vi "struck to array.vi"(10 "Task Info":T1={"Accele Task"=[], "Simulate"=FALSE, "采样率"={"AISampleRate"=10123, "CouplingType"=10000, "Butter"=1000}, "Trig"={"PreTrigCNT"=0, "TriggerMode"=enum."中间触发", "TriggerSource"=enum."软件触发", "ATRTriggerChannel"=enum."通道0", "TriggerDir"=enum."下降沿触发", "TrigLevelVolt"=0.0, "bAvailableTrig"=FALSE}, "clock"={"EN"=FALSE, "clocksource"=enum."内部时钟", "outclocksource"=enum."Trig0"}, "delay(S)"=0.0} {"采样率"."CouplingType" items=["直流耦合", "交流耦合"]}) -> (2 "array":i32[](array[numeric]))   [LabVIEW 2009]
uses:
  Ctrls/Task Info.ctl
  Ctrls/Acceleration Channel Config_Ctrls-某型振动实验台测试系统.ctl
  Ctrls/Sample Information.ctl
  Ctrls/Trig.ctl
  Ctrls/clock.ctl
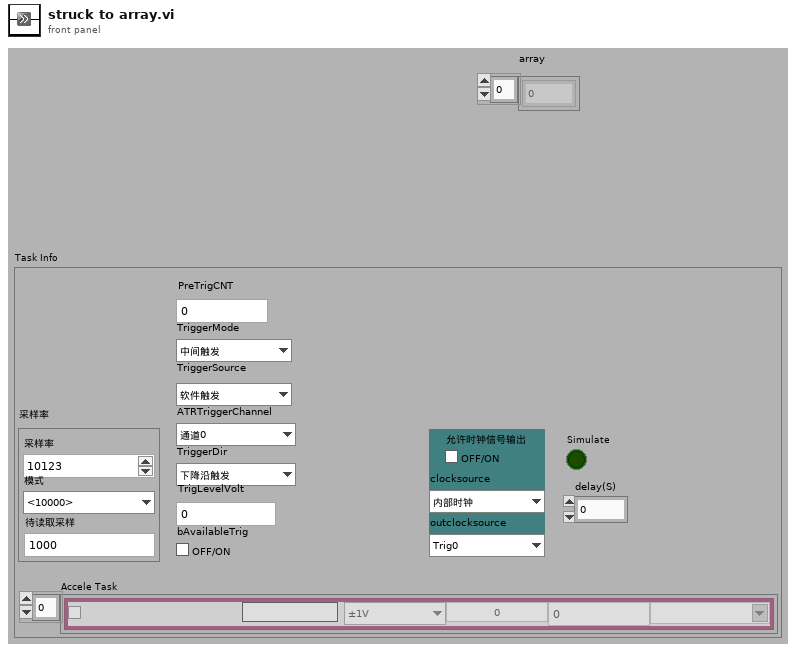
[diagram p1: front panel]
types:
  T1 = typedef "Task Info.ctl" = cluster{"Accele Task":T2[], "Simulate":bool, "采样率":T3, "Trig":T4, "clock":T5, "delay(S)":dbl}
  T2 = typedef "Acceleration Channel Config_Ctrls-某型振动实验台测试系统.ctl" = cluster{"Enable":bool, "Name":string, "range":enum16{"±1V", "±5V"}, "SensValue":dbl, "PhysicalName":string, "off":dbl, "Sensunits":string}
  T3 = typedef "Sample Information.ctl" = cluster{"AISampleRate":i32, "CouplingType":i32, "Butter":i32}
  T4 = typedef "Trig.ctl" = cluster{"PreTrigCNT":i32, "TriggerMode":enum16{"中间触发", "后触发", "预触发", "硬件延时触发"}, "TriggerSource":enum16{"软件触发", "DTR信号源", "ATR信号源", "Triger信号触发"}, "ATRTriggerChannel":enum16{"通道0", "通道1", "通道2", "通道3"}, "TriggerDir":enum16{"下降沿触发", "上升沿触发", "上下边没均触发"}, "TrigLevelVolt":sgl, "bAvailableTrig":bool}
  T5 = typedef "clock.ctl" = cluster{"EN":bool, "clocksource":enum16{"内部时钟", "外部时钟"}, "outclocksource":enum16{"Trig0", "Trig1", "Trig2", "Trig3", "Trig4", "Trig5", "Trig6", "Trig7", "PXI_STAR"}}
  T6 = enum16{"Trig0", "Trig1", "Trig2", "Trig3", "Trig4", "Trig5", "Trig6", "Trig7", "PXI_STAR"}
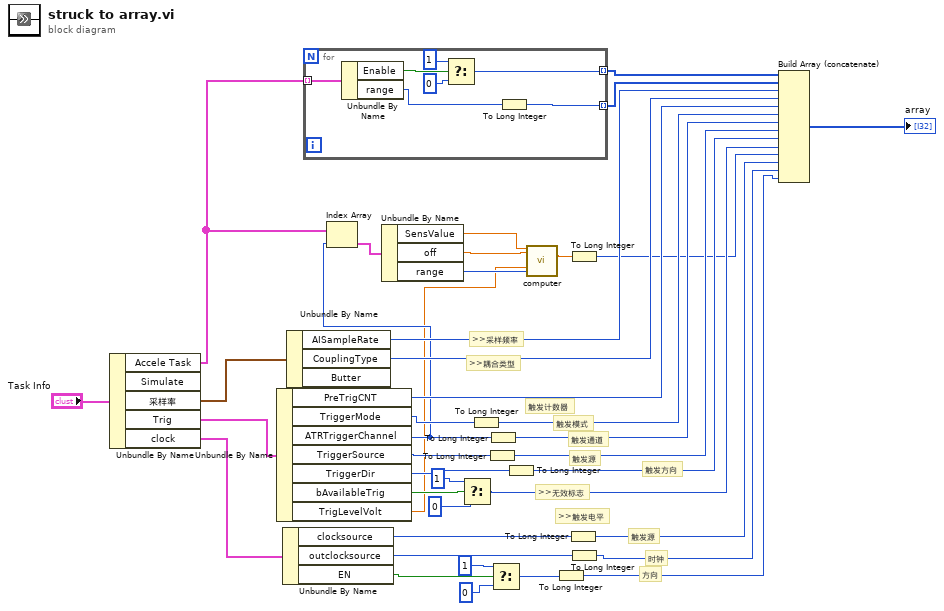
[diagram p0: block diagram]
diagram:
  # "方向"
  # "时钟"
  # "触发源"
  # ">>触发电平"
  # ">>无效标志"
  # "触发方向"
  # "触发源"
  # "触发通道"
  # "触发模式"
  # "触发计数器"
  # ">>耦合类型"
  # ">>采样频率"
  n1 = Unbundle By Name("Task Info") -> ("Accele Task"=w9:T2[], "采样率"=w38:T3, "Trig"=w37:T4, "clock"=w36:T5)  [unwired: 1 out]
  n2 = Unbundle By Name(w37) -> ("PreTrigCNT"=w31:i32, "TriggerMode"=w30:enum16{"中间触发", "后触发", "预触发", "硬件延时触发"}, "ATRTriggerChannel"=w8:enum16{"通道0", "通道1", "通道2", "通道3"}, "TriggerSource"=w18:enum16{"软件触发", "DTR信号源", "ATR信号源", "Triger信号触发"}, "TriggerDir"=w26:enum16{"下降沿触发", "上升沿触发", "上下边没均触发"}, "bAvailableTrig"=w17:bool, "TrigLevelVolt"=w3:sgl)
  n3 = Unbundle By Name(w36) -> ("clocksource"=w11:enum16{"内部时钟", "外部时钟"}, "outclocksource"=w22:T6, "EN"=w13:bool)
  n4 = Unbundle By Name(w38) -> ("AISampleRate"=w32:i32, "CouplingType"=w33:i32)  [unwired: 1 out]
  n5 = for {
    tunnel: w9 -> [w44] mode=indexing
    tunnel: [w42] -> w35 mode=indexing
    tunnel: [w40] -> w34 mode=indexing
    n6 = Unbundle By Name(w44) -> ("Enable"=w43:bool, "range"=w41:enum16{"±1V", "±5V"})
    n7 = Select(t=1, s=w43, f=0) -> (s? t:f=w42:i32)
    n8 = To Long Integer(number=w41) -> (32bit integer=w40:i32)
  }
  n9 = Index Array(array=w9, index=w8) -> (element=w7:T2)
  n10 = Unbundle By Name(w7) -> ("SensValue"=w6:dbl, "off"=w5:dbl, "range"=w4:enum16{"±1V", "±5V"})
  n11 = Select(t=1, s=w17, f=0) -> (s? t:f=w16:i32)
  n12 = To Long Integer(number=w30) -> (32bit integer=w29:i32)
  n13 = To Long Integer(number=w18) -> (32bit integer=w28:i32)
  n14 = To Long Integer(number=w8) -> (32bit integer=w27:i32)
  n15 = Select(t=1, s=w13, f=0) -> (s? t:f=w12:i32)
  n16 = To Long Integer(number=w26) -> (32bit integer=w23:i32)
  n17 = call "computer.vi"("sen"=w6, "off"=w5, "range"=w4, "trig"=w3) -> ("结果"=w2:dbl)  [unwired: 4 in, 7 out]
  n18 = To Long Integer(number=w12) -> (32bit integer=w14:i32)
  n19 = To Long Integer(number=w11) -> (32bit integer=w10:i32)
  n20 = To Long Integer(number=w2) -> (32bit integer=w1:i32)
  n21 = To Long Integer(number=w22) -> (32bit integer=w15:i32)
  n22 = Build Array (concatenate)(w35, w34, w32, w33, w31, w29, w27, w28, w23, w16, w1, w10, w15, w14) -> (→"array":i32[])
